vi "ClassPanel.vi"(8 "error in (no error)":errorcluster caption="entrée d'erreur (pas d'erreur)", 11 "ThorCCS200.lvclass":refnum<class "ThorCCS200.lvclass">) -> (0 "error out":errorcluster caption="sortie d'erreur", 3 "ThorCCS200.lvclass Out":refnum<class "ThorCCS200.lvclass">)   [LabVIEW 2019, in "ThorCCS200.lvclass"]
uses:
  ThorCCS200.lvclass
  C:/Programmes Labview/LabScanV1A/DevicesClass/BaseDevice/BaseDevice.lvclass
  BaseDevice/Accessor/GetClassEvent.vi
panel:
  in  "AcqFromWinCont":bool
  in  "AcqFromWinSgl":bool
  in  "AcqWind":bool
  in  "AquireImage":bool caption="MiseAJour"
  in  "Save Data":bool caption="Save\nData"
  out "AcqTime":dbl caption="Acq. Time (s)" format="%#.3f"
  in  "IntegTime":dbl=10.0 caption="Integration\nTime (ms)" min=0.1 max=100000.0 step=0.1
  out "Aquiring":bool
  in  "MainProgQ":refnum<queue>
  in  "MainProgQEvent":refnum<user-event>
  in  "Acq":bool
  in  "Stop":bool
  out "Init Program":bool
  # "Thor CCS200"
  # "Single Acq"
  # "this MUST labeled with class name"
  # "this MUST be present and labeled \"Stop\" and \"Acq\""
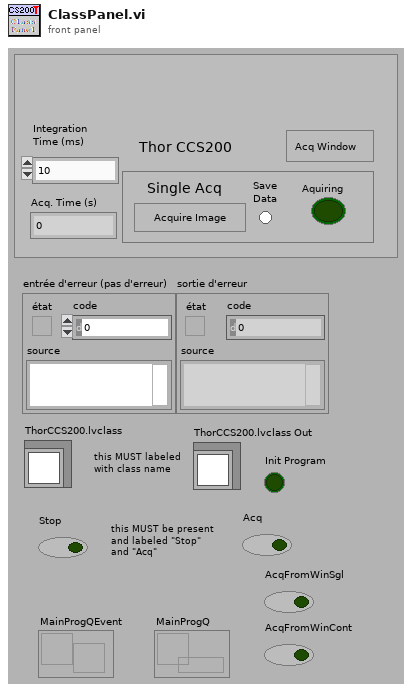
[diagram p1: front panel]
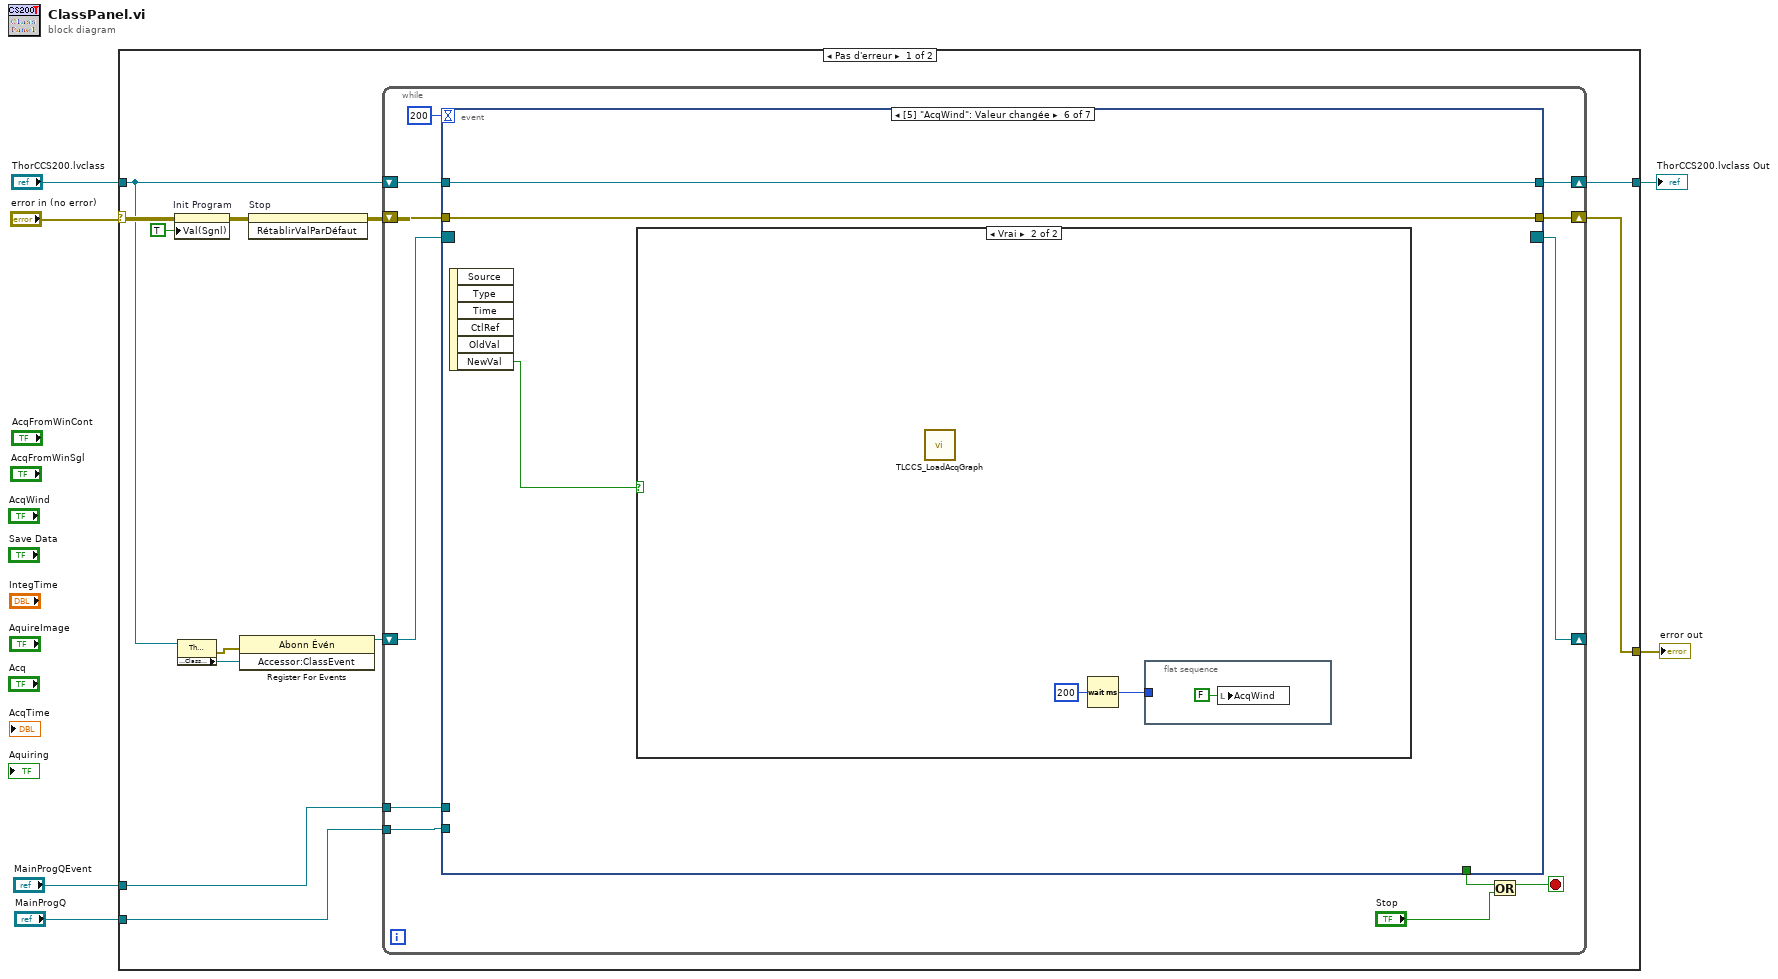
[diagram p0: block diagram]
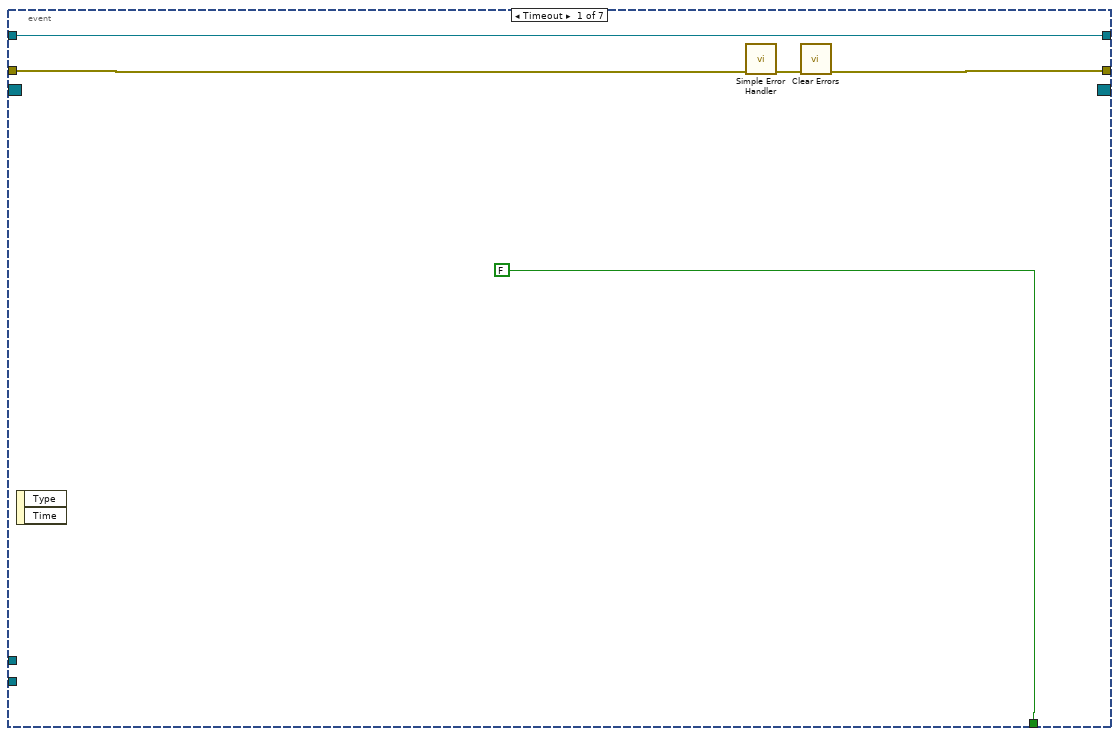
[diagram p2: hidden frame]
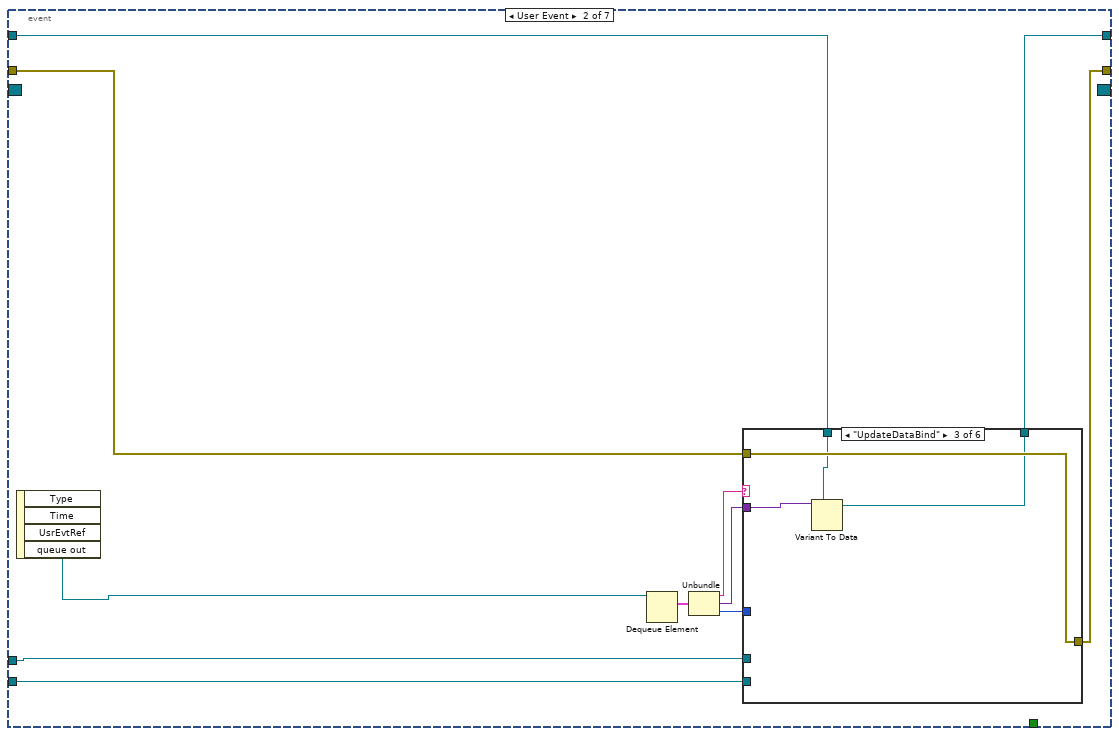
[diagram p3: hidden frame]
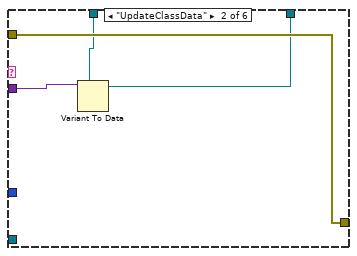
[diagram p5: hidden frame]
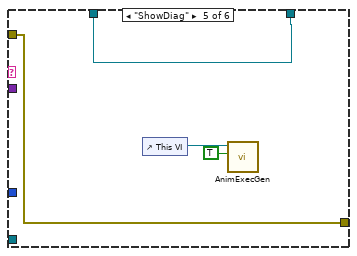
[diagram p7: hidden frame]
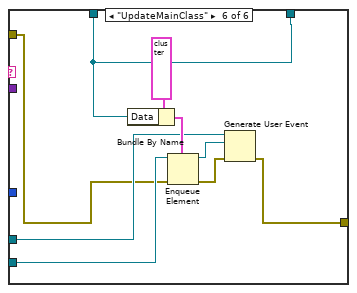
[diagram p8: hidden frame]
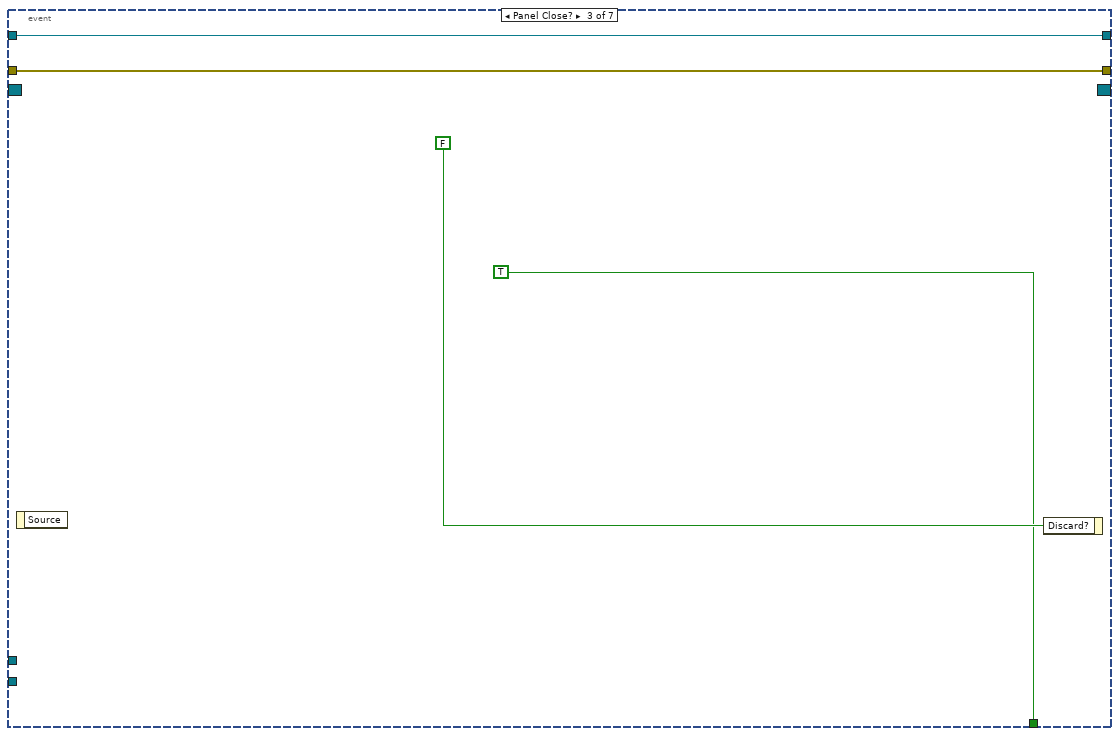
[diagram p9: hidden frame]
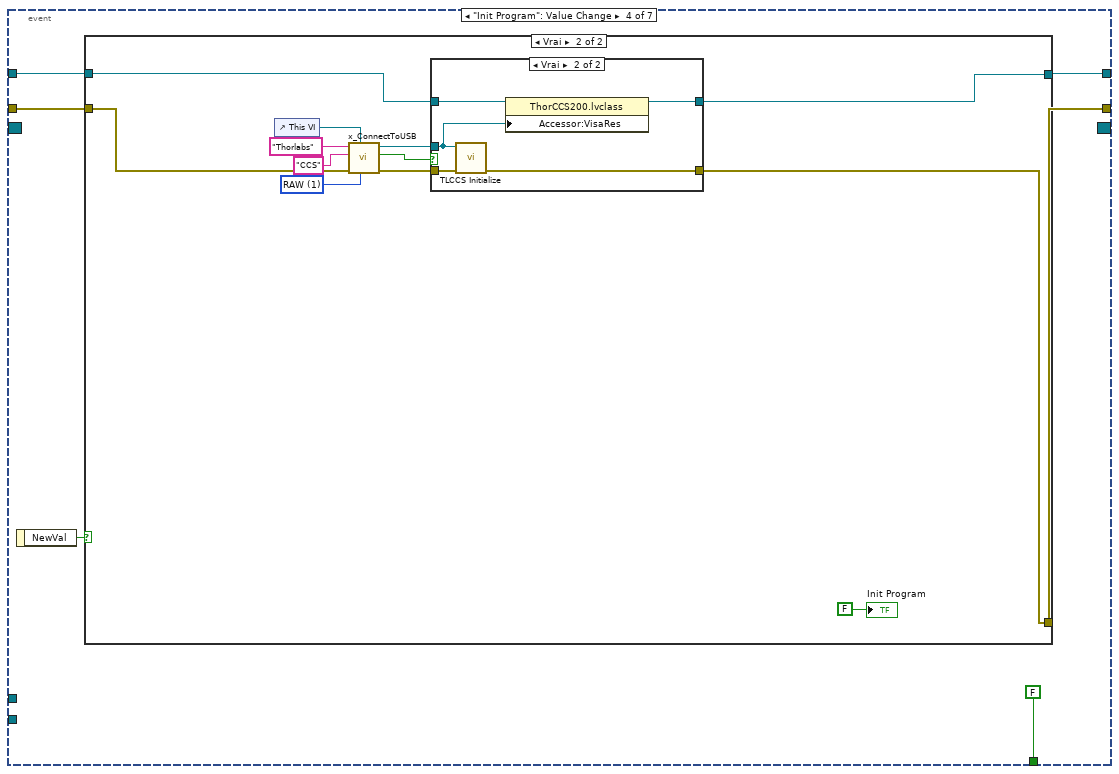
[diagram p10: hidden frame]
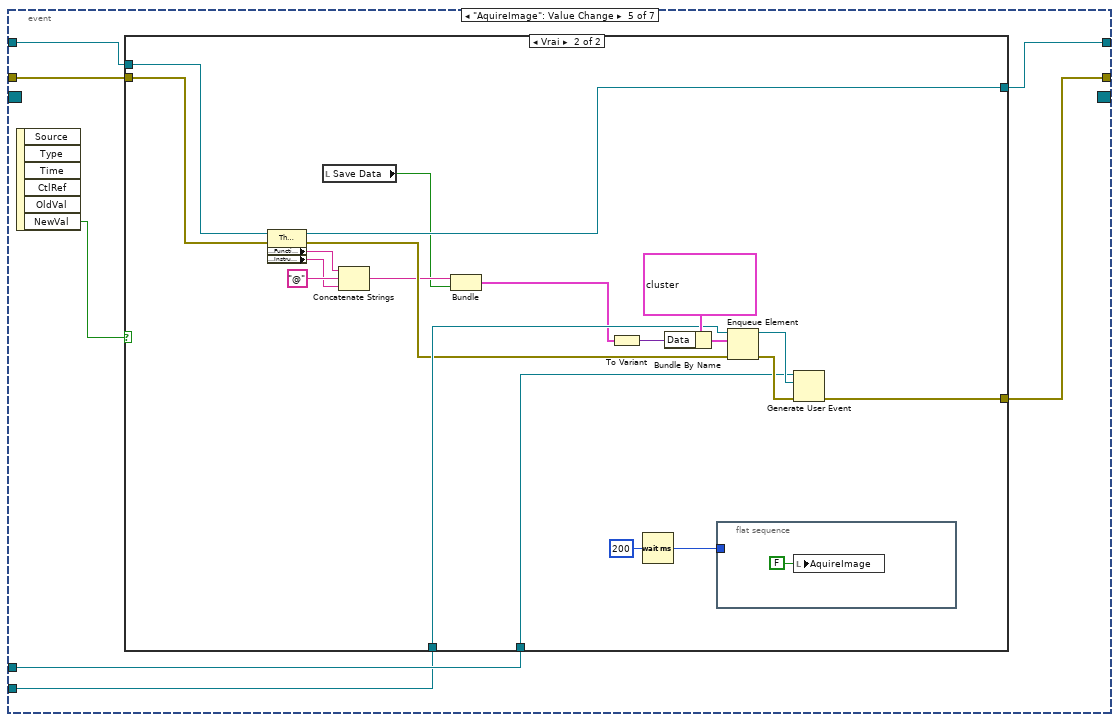
[diagram p13: hidden frame]
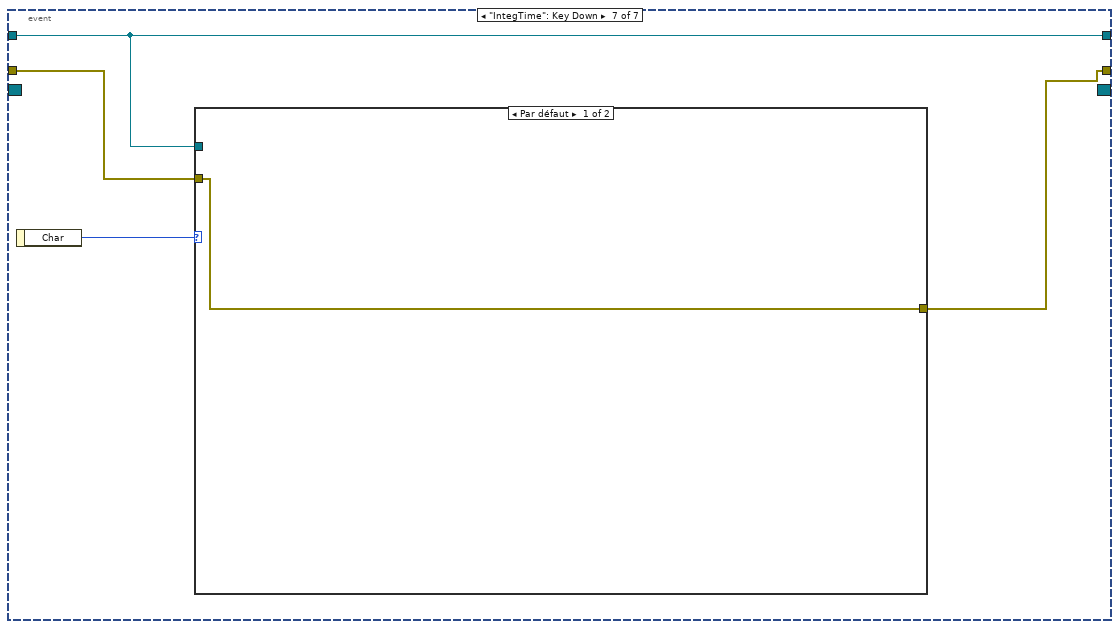
[diagram p16: hidden frame]
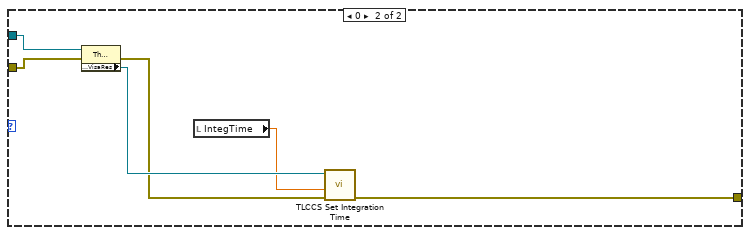
[diagram p17: hidden frame]
diagram:
  n1 = case shown="Pas d'erreur" "error in (no error)" {
    selector: "error in (no error)" -> [w15 w151]
    tunnel: [w18 w151] -> w5
    tunnel: "ThorCCS200.lvclass" -> [w10 w150]
    tunnel: [w16 w150] -> w3
    tunnel: "MainProgQEvent" -> [w8 _]
    tunnel: "MainProgQ" -> [w7 _]
    frame No Error {
      n2 = property on="Init Program" class="Bool (strict)"(error in=w15, "Val(Sgnl)"=TRUE ("Valeur (Signalisation)")) -> (error out=w14:errorcluster)  [unwired: 1 in, 1 out]
      n3 = property class="ThorCCS200.lvclass"(reference=w10) -> (error out=w12:errorcluster, "Accessor:ClassEvent"=w11:refnum<user-event>)  [unwired: 1 in, 1 out]
      n4 = register-events(error in=w12, w11) -> (reference out=w9:refnum<event-registration>)  [unwired: 1 in, 1 out]
      n5 = invoke on="Stop" class="Bool (strict)" method="RétablirValParDéfaut"(error in=w14) -> (error out=w13:errorcluster)  [unwired: 2 in, 2 out]
      n6 = while {
        shift-right: [w28] -> w18
        shift-left: w13 -> [w29]
        shift-right: [w25] -> w16
        shift-left: w10 -> [w27]
        shift-right: [w21] -> _
        shift-left: w9 -> [w22]
        tunnel: w8 -> [w20]
        tunnel: w7 -> [w19]
        stop <- w24 stop-if-true
        n7 = event shown="[5] \"AcqWind\": Valeur changée" {
          selector: w22 -> [_ _ _ _ _ _ _]
          dyn-events: [_ _ _ _ _ _ _] -> w21
          timeout: 200 -> [_ _ _ _ _ _ _]
          tunnel: w29 -> [w33 w45 w73 w80 w108 w134 w141]
          tunnel: [w31 w39 w73 w79 w104 w134 w139] -> w28
          tunnel: w27 -> [w34 w46 w72 w77 w109 w135 w140]
          tunnel: [FALSE _ TRUE FALSE _ _ _] -> w26
          tunnel: [w34 w38 w72 w76 w107 w135 w140] -> w25
          tunnel: w20 -> [_ w37 _ _ w106 _ _]
          tunnel: w19 -> [_ w36 _ _ w105 _ _]
          event Timeout {
            n8 = event-data() -> ()  [unwired: 1 in, 2 out]
            n9 = call <vilib>:"Simple Error Handler.vi"("error in (no error)"=w33) -> ("error out"=w32:errorcluster)  [unwired: 4 in, 4 out]
            n10 = call <vilib>:"Clear Errors.vi"("error in (no error)"=w32) -> ("error out"=w31:errorcluster)  [unwired: 5 in, 1 out]
          }
          event User Event {
            n11 = event-data() -> ("queue out"=w43:refnum<queue>)  [unwired: 1 in, 3 out]
            n12 = Dequeue Element(queue=w43) -> (element=w44:cluster{"Message":string, "Data":variant, i32})  [unwired: 2 in, 3 out]
            n13 = Unbundle(w44) -> ("Message"=w42:string, "Data"=w41:variant, w40:i32)
            n14 = case shown="\"UpdateDataBind\"" w42 {
              tunnel: w45 -> [w48 w52 w56 w57 w61 w64]
              tunnel: w41 -> [_ w51 w55 _ _ _]
              tunnel: w46 -> [w47 w50 w54 w58 w62 w67]
              tunnel: [w47 w49 w53 w58 w62 w67] -> w38
              tunnel: [w48 w52 w56 w57 w61 w63] -> w39
              tunnel: w40 -> [_ _ _ _ _ _]
              tunnel: w37 -> [_ _ _ _ _ w66]
              tunnel: w36 -> [_ _ _ _ _ w65]
              frame Default {
              }
              frame "UpdateClassData" {
                n15 = Variant To Data(type=w50, Variant=w51) -> (data=w49:refnum<class "ThorCCS200.lvclass">)  [unwired: 1 in, 1 out]
              }
              frame "UpdateDataBind" {
                n16 = Variant To Data(type=w54, Variant=w55) -> (data=w53:refnum<class "ThorCCS200.lvclass">)  [unwired: 1 in, 1 out]
              }
              frame "MeasDone" {
              }
              frame "ShowDiag" {
                n17 = control-ref of="This VI"() -> (w60:refnum<vi>)
                n18 = call <userlib>:"AnimExecGen.vi"("Animer l'exécution ?"=TRUE, "ViRef"=w60) -> ()  [unwired: 9 in, 1 out]
              }
              frame "UpdateMainClass" {
                n19 = Bundle By Name(cluster=cluster{"Message":string, "Data":variant, i32} {"Message"="", "Data"=variant, 0} ("élément"), "Data"=w67) -> (w68:cluster{"Message":string, "Data":variant, i32})
                n20 = Enqueue Element(queue=w65, element=w68, error in (no error)=w64) -> (queue out=w71:refnum<queue>, error out=w70:errorcluster)  [unwired: 1 in, 1 out]
                n21 = Generate User Event(user event=w66, event data cluster=w71, error in=w70) -> (error out=w63:errorcluster)  [unwired: 1 in, 1 out]
              }
            }
          }
          event Panel Close? {
            n22 = event-data() -> ()  [unwired: 1 in, 1 out]
            n23 = event-data("Discard?"=FALSE ("Rejeter ?")) -> ()  [unwired: 1 in, 1 out]
          }
          event "Init Program": Value Change {
            n24 = event-data() -> ("NewVal"=w81:bool)  [unwired: 1 in]
            n25 = case shown="Vrai" w81 {
              tunnel: w80 -> [w83 w87]
              tunnel: [w83 w88] -> w79
              tunnel: [w82 w84] -> w76
              tunnel: w77 -> [w82 w85]
              frame False {
              }
              frame True {
                w91 = u16 1 items=["INSTR", "RAW"] ("Instrument Class")
                n26 = control-ref of="This VI"() -> (w92:refnum<vi>)
                n27 = call <instrlib>:"x_ConnectToUSB.vi"("Instrument Class"=w91, "VI reference"=w92, "error in"=w87, "Model"="CCS", "Manufacturer"="Thorlabs") -> ("error out"=w90:errorcluster, "FoundUSB"=w89:bool, "USB Ref"=w86:refnum<visa-resource-name>)  [unwired: 4 in]
                n28 = case shown="Vrai" w89 {
                  tunnel: w90 -> [w97 w102]
                  tunnel: w86 -> [_ w99]
                  tunnel: [w97 w101] -> w88
                  tunnel: w85 -> [w96 w100]
                  tunnel: [w96 w98] -> w84
                  frame False {
                  }
                  frame True {
                    n29 = call <instrlib>:"TLCCS Initialize.vi"("error in (no error)"=w102, "resource name"=w99) -> ("error out"=w101:errorcluster)  [unwired: 8 in, 1 out]
                    n30 = property class="ThorCCS200.lvclass"(reference=w100, "Accessor:VisaRes"=w99) -> (reference out=w98:refnum<class "ThorCCS200.lvclass">)  [unwired: 1 in, 1 out]
                  }
                }
                "Init Program" <- FALSE
              }
            }
          }
          event "AquireImage": Value Change {
            n31 = event-data() -> ("NewVal"=w103:bool)  [unwired: 1 in, 5 out]
            n32 = case shown="Vrai" w103 {
              tunnel: w109 -> [w111 w118]
              tunnel: w108 -> [w110 w117]
              tunnel: [w111 w116] -> w107
              tunnel: w106 -> [_ w119]
              tunnel: w105 -> [_ w123]
              tunnel: [w110 w112] -> w104
              frame False {
              }
              frame True {
                n33 = property class="ThorCCS200.lvclass"(reference=w118, error in=w117) -> (reference out=w116:refnum<class "ThorCCS200.lvclass">, error out=w122:errorcluster, "Accessor:Function"=w126:string, "Accessor:InstrumentName"=w124:string)
                n34 = local read "Save Data"() -> (w115:bool)
                n35 = Concatenate Strings(w126, "@" ("chaîne"), w124) -> (w120:string)
                n36 = Bundle(w120, "Save Data"=w115) -> (w121:cluster{string, "Save Data":bool})  [unwired: 1 in]
                n37 = To Variant(anything=w121) -> (Variant=w129:variant)
                n38 = Wait (ms)(milliseconds to wait=u32 200 ("attente (ms)")) -> (millisecond timer value=w113:u32)
                n39 = Bundle By Name(cluster=cluster{"Message":string, "Data":variant, i32} {"Message"="ArrayDevAcqSetup", "Data"=variant, 0} ("élément"), "Data"=w129) -> (w128:cluster{"Message":string, "Data":variant, i32})
                n40 = flat-sequence {
                  tunnel: w113 -> [_]
                  frame #0 {
                    n41 = local write "AquireImage"(FALSE ("AquireImage")) -> ()
                  }
                }
                n42 = Enqueue Element(queue=w123, element=w128, error in (no error)=w122) -> (queue out=w131:refnum<queue>, error out=w127:errorcluster)  [unwired: 1 in, 1 out]
                n43 = Generate User Event(user event=w119, event data cluster=w131, error in=w127) -> (error out=w112:errorcluster)  [unwired: 1 in, 1 out]
              }
            }
          }
          event "AcqWind": Value Change {
            n44 = event-data() -> ("NewVal"=w133:bool)  [unwired: 1 in, 5 out]
            n45 = case shown="Vrai" w133 {
              frame False {
              }
              frame True {
                n46 = call <instrlib>:"TLCCS_LoadAcqGraph.vi"() -> ()  [unwired: 6 in, 6 out]
                n47 = Wait (ms)(milliseconds to wait=u32 200 ("attente (ms)")) -> (millisecond timer value=w137:u32)
                n48 = flat-sequence {
                  tunnel: w137 -> [_]
                  frame #0 {
                    n49 = local write "AcqWind"(FALSE ("ContAcq")) -> ()
                  }
                }
              }
            }
          }
          event "IntegTime": Key Down {
            n50 = event-data() -> ("Char"=w142:i16)  [unwired: 1 in]
            n51 = case shown="Par défaut" w142 {
              tunnel: w140 -> [_ w149]
              tunnel: w141 -> [w143 w148]
              tunnel: [w143 w144] -> w139
              frame Default {
              }
              frame 0 {
                n52 = property class="ThorCCS200.lvclass"(reference=w149, error in=w148) -> (error out=w146:errorcluster, "Accessor:VisaRes"=w147:refnum<visa-resource-name>)  [unwired: 1 out]
                n53 = local read "IntegTime"() -> (w145:dbl)
                n54 = call <instrlib>:"TLCCS Set Integration Time.vi"("error in (no error)"=w146, "Integration Time [s] (0.001)"=w145, "instrument handle"=w147) -> ("error out"=w144:errorcluster)  [unwired: 7 in, 1 out]
              }
            }
          }
        }
        n55 = Or(x=w26, y="Stop") -> (x .or. y?=w24:bool)
      }
    }
    frame Error {
    }
  }
  "error out" <- w5
  "ThorCCS200.lvclass Out" <- w3
